vi "PH_VacuumControl.Show MultiTrend.vi"(0 "i ref in":refnum<vi>, 5 "error in":errorcluster) -> (14 "i ref out":refnum<vi>, 19 "error out":errorcluster)   [LabVIEW 2014, in "PH_VacuumControl.lvlib"]
doc: "This VI shows the Multi Trend data."
uses:
  PH_VacuumControl.lvlib
  <vilib>/Utility/miscctls.llb/LVCursorListTypeDef.ctl
panel:
  in  "Cursor List":T1
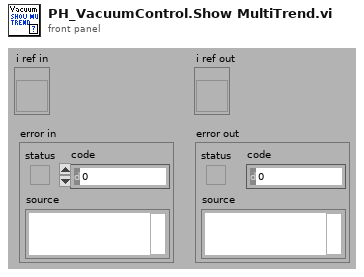
[diagram p1: front panel]
types:
  T1 = typedef "LVCursorListTypeDef.ctl" = cluster{"Name":string, "Color":u32, "Style":u8, "Point Style":u8, "Name Visible":bool, "Allow Drag":bool, "Cursor Mode":u32, "Plot":i32, "Index":i32, "Position":cluster{"X":dbl, "Y":dbl}, "X Scale":u32, "Y Scale":u32, "Watch Plots":i32[], "Watch All Plots":bool, "Plot Area":i32, "Label Offset":cluster{"X":dbl, "Y":dbl}}[]
  T2 = typedef "PH_VacuumControl.lvlib/PH_VacuumControl.i attribute.ctl" = cluster{"GUI Refs":cluster{"Exit":refnum<vi>, "Set Unit":refnum<vi>, "Device found":refnum<vi>, "Busy":refnum<vi>, "State":refnum<vi>, "Delete":refnum<vi>, "Channels":refnum<vi>, "Channel Name":refnum<vi>, "Trend":refnum<vi>, "Logarithmic":refnum<vi>, "Limit reached":refnum<vi>, "Channel Name 1 MT":refnum<vi>, "Channel Name 2 MT":refnum<vi>, "Trend MT":refnum<vi>, "Logarithmic MT":refnum<vi>, "Limit reached MT":refnum<vi>}, "Device found":bool, "Busy":bool, "Selected Unit":i32, "Channels [mbar]":T3, "Channel Names":cluster{"Channel 1":string, "Channel 2":string, "Channel 3":string, "Channel 4":string, "Channel 5":string, "Channel 6":string}, "Status":T4, "AGCxxx VISA Cluster":T5, "Instr Firmware Revision":string, "Service IDs Pressure":cluster{"Channel 1":i32, "Channel 2":i32, "Channel 3":i32, "Channel 4":i32, "Channel 5":i32, "Channel 6":i32}, "Service IDs Limits":cluster{"Channel 1":i32, "Channel 2":i32, "Channel 3":i32, "Channel 4":i32, "Channel 5":i32, "Channel 6":i32}, "Trend":cluster{"Start Point":timestamp, "Pressures [mbar] Channel 1":dbl[], "Pressures [mbar] Channel 2":dbl[], "Pressures [mbar] Channel 3":dbl[], "Pressures [mbar] Channel 4":dbl[], "Pressures [mbar] Channel 5":dbl[], "Pressures [mbar] Channel 6":dbl[], "Timebase [s]":i32[], "Trend Channel":u16, "Start Fit":dbl, "Trend Channel 1 MT":u16, "Trend Channel 2 MT":u16, "Start or continue Fit MT":dbl, "Continue or start Fit MT":dbl, "Datasets strored":i32, "Dataarray Size":i32}, "Running":bool}
  T3 = typedef "PH_VacuumControl.lvlib/PH_VacuumControl.Channels.ctl" = cluster{"Channel 1":dbl, "Channel 2":dbl, "Channel 3":dbl, "Channel 4":dbl, "Channel 5":dbl, "Channel 6":dbl, "Name Channel 1":string, "Name Channel 2":string, "Name Channel 3":string, "Name Channel 4":string, "Name Channel 5":string, "Name Channel 6":string, "Upper Limit":dbl, "Upper Limit 2":dbl, "Upper Limit 3":dbl, "Upper Limit 4":dbl, "Upper Limit 5":dbl, "Upper Limit 6":dbl}
  T4 = typedef "PH_StatusHandler.lvlib/PH_StatusHandler.Status.ctl" = i16
  T5 = typedef "AGCxxx - Driver.lvlib/AGCxxx VISA Control.ctl" = cluster{"VISA resource name":refnum<visa-resource-name>, "VISA Timeout Value (1000 ms)":u32, "Lock Timeout (1000 ms)":u32, "MAX Channel (6)":i32}
  T6 = cluster{"Name":string, "Color":u32, "Style":u8, "Point Style":u8, "Name Visible":bool, "Allow Drag":bool, "Cursor Mode":u32, "Plot":i32, "Index":i32, "Position":cluster{"X":dbl, "Y":dbl}, "X Scale":u32, "Y Scale":u32, "Watch Plots":i32[], "Watch All Plots":bool, "Plot Area":i32, "Label Offset":cluster{"X":dbl, "Y":dbl}}
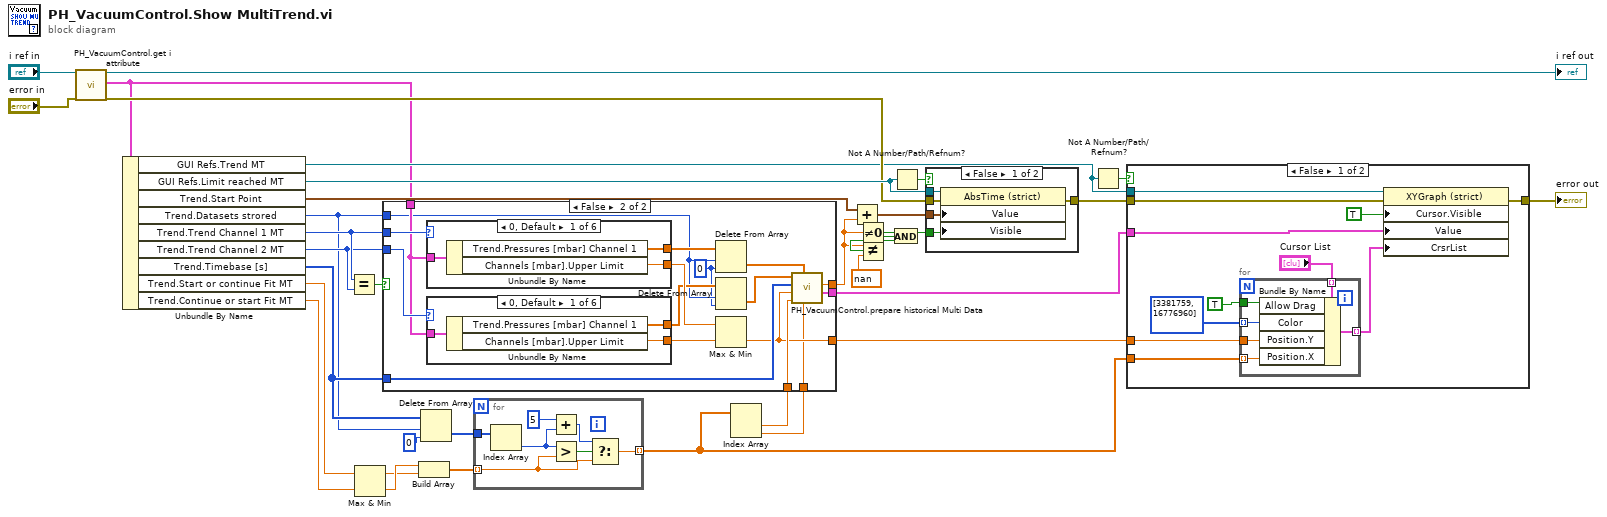
[diagram p0: block diagram]
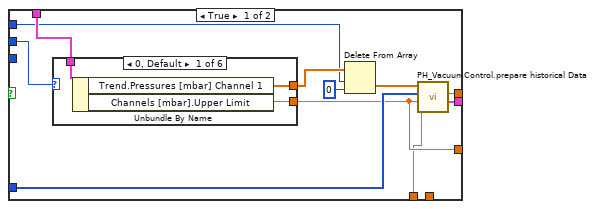
[diagram p2: hidden frame]
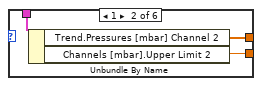
[diagram p3: hidden frame]
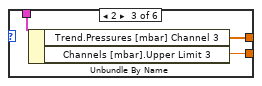
[diagram p4: hidden frame]
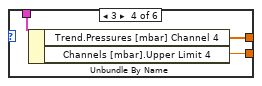
[diagram p5: hidden frame]
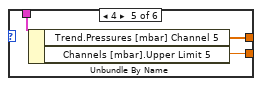
[diagram p6: hidden frame]
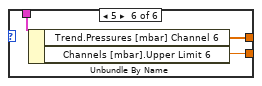
[diagram p7: hidden frame]
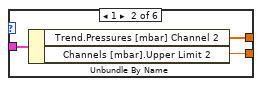
[diagram p8: hidden frame]
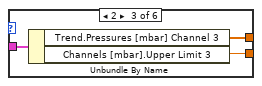
[diagram p9: hidden frame]
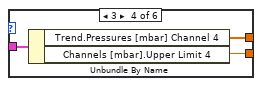
[diagram p10: hidden frame]
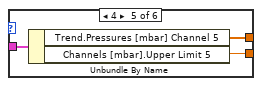
[diagram p11: hidden frame]
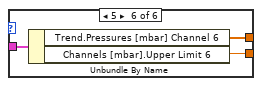
[diagram p12: hidden frame]
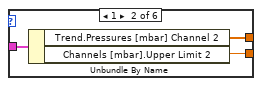
[diagram p13: hidden frame]
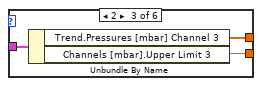
[diagram p14: hidden frame]
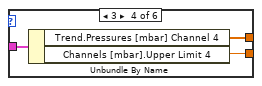
[diagram p15: hidden frame]
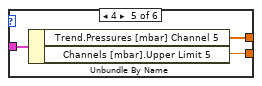
[diagram p16: hidden frame]
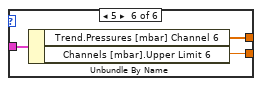
[diagram p17: hidden frame]
diagram:
  n1 = call "PH_VacuumControl.get i attribute.vi"("i ref in"="i ref in", "error in (no error)"="error in") -> ("i ref out"=→"i ref out":refnum<vi>, "i attribute"=w29:T2, "error out"=w33:errorcluster)  [unwired: 15 in]
  n2 = Unbundle By Name(w29) -> ("GUI Refs.Trend MT"=w32:refnum<vi>, "GUI Refs.Limit reached MT"=w34:refnum<vi>, "Trend.Start Point"=w35:timestamp, "Trend.Datasets strored"=w1:i32, "Trend.Trend Channel 1 MT"=w22:u16, "Trend.Trend Channel 2 MT"=w6:u16, "Trend.Timebase [s]"=w31:i32[], "Trend.Start or continue Fit MT"=w24:dbl, "Trend.Continue or start Fit MT"=w23:dbl)
  n3 = Equal?(x=w22, y=w6) -> (x = y?=w7:bool)
  n4 = Max & Min(x=w24, y=w23) -> (max(x,y)=w21:dbl, min(x,y)=w25:dbl)
  n5 = Build Array(w25, w21) -> (w9:dbl[])
  n6 = Delete From Array(array=w31, length=w1, index=0) -> (deleted portion=w3:i32[])  [unwired: 1 out]
  n7 = for {
    tunnel: [w39] -> w5 mode=indexing
    tunnel: w3 -> [w37]
    tunnel: w9 -> [w36] mode=indexing
    n8 = Index Array(array=w37) -> (element=w40:i32)  [unwired: 1 in]
    n9 = Add(x=5, y=w40) -> (x+y=w42:i32)
    n10 = Greater?(x=w40, y=w36) -> (0:w38:bool)
    n11 = Select(t=w42, s=w38, f=w36) -> (s? t:f=w39:dbl)
  }
  n12 = Index Array(array=w5) -> (element #1=w8:dbl, element #2=w4:dbl)  [unwired: 2 in]
  n13 = case shown="False" w7 {
    tunnel: w31 -> [w53 w88]
    tunnel: w29 -> [w52 w79]
    tunnel: w22 -> [w51 w87]
    tunnel: [w50 w86] -> w17
    tunnel: [w49 w81] -> w12
    tunnel: [w48 w85] -> w10
    tunnel: w8 -> [w47 w84]
    tunnel: w6 -> [_ w83]
    tunnel: w4 -> [_ w78]
    tunnel: w1 -> [w44 w73]
    frame True {
      n14 = case shown="0, Default" w51 {
        tunnel: w52 -> [w56 w59 w62 w65 w68 w71]
        tunnel: [w55 w58 w61 w64 w67 w70] -> w45
        tunnel: [w54 w57 w60 w63 w66 w69] -> w49
        frame 0, Default {
          n15 = Unbundle By Name(w56) -> ("Trend.Pressures [mbar] Channel 1"=w55:dbl[], "Channels [mbar].Upper Limit"=w54:dbl)
        }
        frame 1 {
          n16 = Unbundle By Name(w59) -> ("Trend.Pressures [mbar] Channel 2"=w58:dbl[], "Channels [mbar].Upper Limit 2"=w57:dbl)
        }
        frame 2 {
          n17 = Unbundle By Name(w62) -> ("Trend.Pressures [mbar] Channel 3"=w61:dbl[], "Channels [mbar].Upper Limit 3"=w60:dbl)
        }
        frame 3 {
          n18 = Unbundle By Name(w65) -> ("Trend.Pressures [mbar] Channel 4"=w64:dbl[], "Channels [mbar].Upper Limit 4"=w63:dbl)
        }
        frame 4 {
          n19 = Unbundle By Name(w68) -> ("Trend.Pressures [mbar] Channel 5"=w67:dbl[], "Channels [mbar].Upper Limit 5"=w66:dbl)
        }
        frame 5 {
          n20 = Unbundle By Name(w71) -> ("Trend.Pressures [mbar] Channel 6"=w70:dbl[], "Channels [mbar].Upper Limit 6"=w69:dbl)
        }
      }
      n21 = Delete From Array(array=w45, length=w44, index=0) -> (deleted portion=w46:dbl[])  [unwired: 1 out]
      n22 = call "PH_VacuumControl.prepare historical Data.vi"("Start Fit"=w47, "Limit"=w49, "Timebase [s]"=w53, "Pressure [mbar]"=w46) -> ("Trend"=w48:cluster{i32[], "Data":dbl[]}[], "Time to reach Limit"=w50:dbl)  [unwired: 5 in]
    }
    frame False {
      w72 = 0 ("index")
      n23 = case shown="0, Default" w87 {
        tunnel: w79 -> [w109 w112 w115 w118 w121 w124]
        tunnel: [w108 w111 w114 w117 w120 w123] -> w76
        tunnel: [w107 w110 w113 w116 w119 w122] -> w80
        frame 0, Default {
          n24 = Unbundle By Name(w109) -> ("Trend.Pressures [mbar] Channel 1"=w108:dbl[], "Channels [mbar].Upper Limit"=w107:dbl)
        }
        frame 1 {
          n25 = Unbundle By Name(w112) -> ("Trend.Pressures [mbar] Channel 2"=w111:dbl[], "Channels [mbar].Upper Limit 2"=w110:dbl)
        }
        frame 2 {
          n26 = Unbundle By Name(w115) -> ("Trend.Pressures [mbar] Channel 3"=w114:dbl[], "Channels [mbar].Upper Limit 3"=w113:dbl)
        }
        frame 3 {
          n27 = Unbundle By Name(w118) -> ("Trend.Pressures [mbar] Channel 4"=w117:dbl[], "Channels [mbar].Upper Limit 4"=w116:dbl)
        }
        frame 4 {
          n28 = Unbundle By Name(w121) -> ("Trend.Pressures [mbar] Channel 5"=w120:dbl[], "Channels [mbar].Upper Limit 5"=w119:dbl)
        }
        frame 5 {
          n29 = Unbundle By Name(w124) -> ("Trend.Pressures [mbar] Channel 6"=w123:dbl[], "Channels [mbar].Upper Limit 6"=w122:dbl)
        }
      }
      n30 = case shown="0, Default" w83 {
        tunnel: w79 -> [w91 w94 w97 w100 w103 w106]
        tunnel: [w90 w93 w96 w99 w102 w105] -> w74
        tunnel: [w89 w92 w95 w98 w101 w104] -> w82
        frame 0, Default {
          n31 = Unbundle By Name(w91) -> ("Trend.Pressures [mbar] Channel 1"=w90:dbl[], "Channels [mbar].Upper Limit"=w89:dbl)
        }
        frame 1 {
          n32 = Unbundle By Name(w94) -> ("Trend.Pressures [mbar] Channel 2"=w93:dbl[], "Channels [mbar].Upper Limit 2"=w92:dbl)
        }
        frame 2 {
          n33 = Unbundle By Name(w97) -> ("Trend.Pressures [mbar] Channel 3"=w96:dbl[], "Channels [mbar].Upper Limit 3"=w95:dbl)
        }
        frame 3 {
          n34 = Unbundle By Name(w100) -> ("Trend.Pressures [mbar] Channel 4"=w99:dbl[], "Channels [mbar].Upper Limit 4"=w98:dbl)
        }
        frame 4 {
          n35 = Unbundle By Name(w103) -> ("Trend.Pressures [mbar] Channel 5"=w102:dbl[], "Channels [mbar].Upper Limit 5"=w101:dbl)
        }
        frame 5 {
          n36 = Unbundle By Name(w106) -> ("Trend.Pressures [mbar] Channel 6"=w105:dbl[], "Channels [mbar].Upper Limit 6"=w104:dbl)
        }
      }
      n37 = Delete From Array(array=w76, length=w73, index=w72) -> (deleted portion=w77:dbl[])  [unwired: 1 out]
      n38 = Delete From Array(array=w74, length=w73, index=w72) -> (deleted portion=w75:dbl[])  [unwired: 1 out]
      n39 = Max & Min(x=w80, y=w82) -> (min(x,y)=w81:dbl)  [unwired: 1 out]
      n40 = call "PH_VacuumControl.prepare historical Multi Data.vi"("Continue Fit"=w78, "Pressure Data 1 [mbar]"=w77, "Start Fit"=w84, "Limit"=w81, "Timebase [s]"=w88, "Pressure Data 2 [mbar]"=w75) -> ("Trend"=w85:cluster{i32[], "Data":dbl[]}[], "Time to reach Limit"=w86:dbl)  [unwired: 3 in]
    }
  }
  n41 = Add(x=w35, y=w17) -> (x+y=w16:timestamp)
  n42 = Not Equal To 0?(x=w17) -> (x != 0?=w15:bool)
  n43 = Not Equal?(x=w17, y=nan) -> (x != y?=w20:bool)
  n44 = And(x=w15, y=w20) -> (x .and. y?=w19:bool)
  n45 = Not A Number/Path/Refnum?(number/path/refnum=w34) -> (NaN/Path/Refnum?=w13:bool)
  n46 = case shown="False" w13 {
    tunnel: w33 -> [w129 w130]
    tunnel: [w128 w130] -> w14
    tunnel: w34 -> [w127 _]
    tunnel: w16 -> [w126 _]
    tunnel: w19 -> [w125 _]
    frame False {
      n47 = property class="AbsTime (strict)"(reference=w127, error in=w129, "Value"=w126, "Visible"=w125) -> (error out=w128:errorcluster)  [unwired: 1 out]
    }
    frame True {
    }
  }
  n48 = Not A Number/Path/Refnum?(number/path/refnum=w32) -> (NaN/Path/Refnum?=w11:bool)
  n49 = case shown="False" w11 {
    tunnel: w14 -> [w141 w148]
    tunnel: [w137 w148] -> w30
    tunnel: w32 -> [w140 _]
    tunnel: w10 -> [w139 _]
    tunnel: w12 -> [w134 _]
    tunnel: w5 -> [w135 _]
    frame False {
      n50 = for {
        tunnel: "Cursor List" -> [w147] mode=indexing
        tunnel: [w146] -> w136 mode=indexing
        tunnel: w135 -> [w145] mode=indexing
        tunnel: w134 -> [w144]
        tunnel: u32[] [3381759, 16776960] -> [w143] mode=indexing
        tunnel: TRUE ("Cursor.Allow Drag") -> [w142]
        n51 = Bundle By Name(cluster=w147, "Allow Drag"=w142, "Color"=w143, "Position.Y"=w144, "Position.X"=w145) -> (w146:T6)
      }
      n52 = property class="XYGraph (strict)"(reference=w140, error in=w141, "Cursor.Visible"=TRUE ("Cursor.Allow Drag"), "Value"=w139, "CrsrList"=w136) -> (error out=w137:errorcluster)  [unwired: 1 out]
    }
    frame True {
    }
  }
  "error out" <- w30
